vi "NPC3SG Live Control.vi"(1 "Running":refnum<vi>, 3 "Drive Live Controls":T1={"Snapshot"=FALSE, "Move Step"=0.5, "Move Home"=FALSE, "Move Down"=FALSE, "Move Up"=FALSE, "Move Left"=FALSE, "Move Right"=FALSE, "Move Out"=FALSE, "Move In"=FALSE} {"Move Step" min=0.0 max=30.0 step=0.1 format="%.3f"}, 4 "Drive Visa Name":refnum<visa-resource-name>="COM5") -> (0 "Reset Switches":bool)   [LabVIEW 2010]
uses:
  TypeDefs/NPC3SG Live Controls.ctl
panel:
  in  "Home":dbl=10.0 format="%.3f"
  # "XY"
  # "Z"
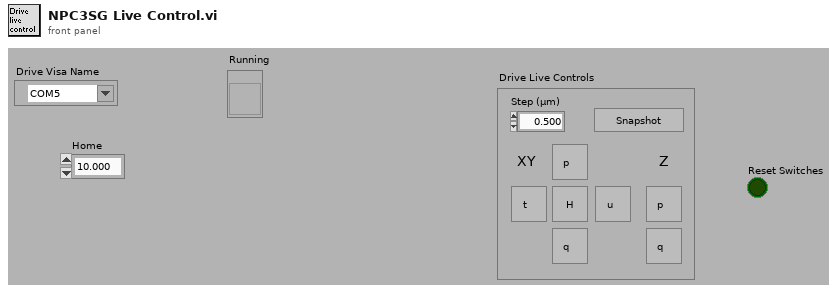
[diagram p1: front panel]
types:
  T1 = typedef "NPC3SG Live Controls.ctl" = cluster{"Snapshot":bool, "Move Step":dbl, "Move Home":bool, "Move Down":bool, "Move Up":bool, "Move Left":bool, "Move Right":bool, "Move Out":bool, "Move In":bool}
  T2 = typedef "NPC3SG Current Values.ctl" = cluster{"Drive X Position":dbl, "Drive Y Position":dbl, "Drive Z Position":dbl}
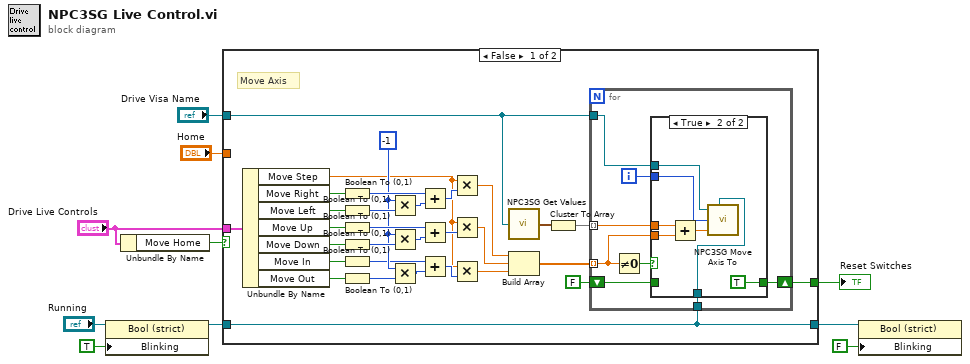
[diagram p0: block diagram]
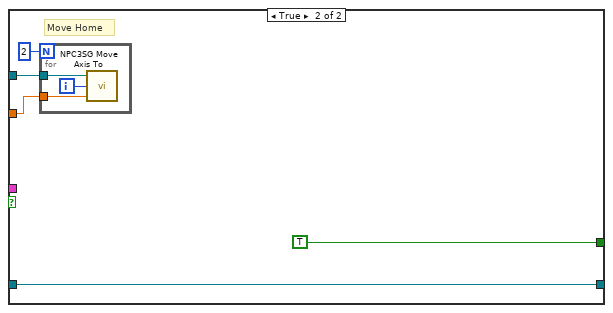
[diagram p3: hidden frame]
diagram:
  n1 = property class="Bool (strict)"(reference="Running", "Blinking"=TRUE ("Blinkend")) -> (reference out=w3:refnum<vi>)  [unwired: 1 in, 1 out]
  n2 = Unbundle By Name("Drive Live Controls") -> ("Move Home"=w8:bool)
  n3 = case shown="False" w8 {
    tunnel: "Drive Visa Name" -> [w16 w61]
    tunnel: [w13 TRUE ("Reset Switches")] -> w10
    tunnel: w3 -> [w11 w59]
    tunnel: "Drive Live Controls" -> [w17 _]
    tunnel: "Home" -> [_ w60]
    tunnel: [w11 w59] -> w1
    frame False {
      w29 = -1
      # "Move Axis"
      n4 = Unbundle By Name(w17) -> ("Move Step"=w18:dbl, "Move Right"=w19:bool, "Move Left"=w24:bool, "Move Up"=w23:bool, "Move Down"=w22:bool, "Move In"=w21:bool, "Move Out"=w20:bool)
      n5 = Boolean To (0,1)(Boolean=w19) -> (0, 1=w33:i16)
      n6 = Boolean To (0,1)(Boolean=w24) -> (0, 1=w31:i16)
      n7 = Boolean To (0,1)(Boolean=w23) -> (0, 1=w35:i16)
      n8 = Boolean To (0,1)(Boolean=w22) -> (0, 1=w32:i16)
      n9 = Boolean To (0,1)(Boolean=w21) -> (0, 1=w27:i16)
      n10 = Boolean To (0,1)(Boolean=w20) -> (0, 1=w30:i16)
      n11 = Multiply(x=w29, y=w31) -> (x*y=w34:i32)
      n12 = Multiply(x=w29, y=w32) -> (x*y=w36:i32)
      n13 = Multiply(x=w29, y=w30) -> (x*y=w28:i32)
      n14 = Add(x=w33, y=w34) -> (x+y=w37:i32)
      n15 = Add(x=w35, y=w36) -> (x+y=w38:i32)
      n16 = Add(x=w27, y=w28) -> (x+y=w26:i32)
      n17 = Multiply(x=w18, y=w37) -> (x*y=w39:dbl)
      n18 = Multiply(x=w18, y=w38) -> (x*y=w40:dbl)
      n19 = Multiply(x=w18, y=w26) -> (x*y=w25:dbl)
      n20 = call "NPC3SG Get Values.vi"("Drive Visa Name"=w16) -> ("Drive Current Values"=w15:T2)
      n21 = Build Array(w39, w40, w25) -> (w41:dbl[])
      n22 = Cluster To Array(cluster=w15) -> (array=w14:dbl[])
      n23 = for {
        tunnel: w41 -> [w48] mode=indexing
        tunnel: w16 -> [w49]
        tunnel: w14 -> [w43] mode=indexing
        shift-right: [w45] -> w13
        shift-left: FALSE ("Reset Switches") -> [w44]
        tunnel: w11 -> [w42]
        i -> [w46]
        n24 = Not Equal To 0?(x=w48) -> (x != 0?=w47:bool)
        n25 = case shown="True" w47 {
          tunnel: w48 -> [_ w54]
          tunnel: w49 -> [_ w57]
          tunnel: w46 -> [_ w56]
          tunnel: [w50 TRUE ("Reset Switches")] -> w45
          tunnel: w44 -> [w50 _]
          tunnel: w43 -> [_ w53]
          tunnel: w42 -> [_ w51]
          frame False {
          }
          frame True {
            n26 = Add(x=w53, y=w54) -> (x+y=w52:dbl)
            n27 = call "NPC3SG Move Axis To.vi"("Drive Visa Name"=w57, "Running"=w51, "Axis"=w56, "Drive Set"=w52) -> ()  [unwired: 3 in, 1 out]
          }
        }
      }
    }
    frame True {
      # "Move Home"
      n28 = for {
        N: 2 -> [_]
        tunnel: w61 -> [w65]
        tunnel: w60 -> [w63]
        i -> [w64]
        n29 = call "NPC3SG Move Axis To.vi"("Drive Visa Name"=w65, "Axis"=w64, "Drive Set"=w63) -> ()  [unwired: 4 in, 1 out]
      }
    }
  }
  "Reset Switches" <- w10
  n30 = property class="Bool (strict)"(reference=w1, "Blinking"=FALSE ("Blinkend")) -> ()  [unwired: 1 in, 2 out]
